vi "InvertedCalculationProjectionAngleOffset.vi"(6 "Y offset":dbl, 7 "X offset":dbl, 8 "RangeX":dbl, 9 "Angle":dbl, 10 "Height":dbl) -> (3 "Width":dbl)   [LabVIEW 2016]
panel:
  out "ResultX":dbl
  out "ResultY":dbl
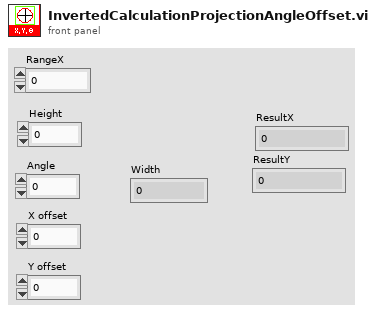
[diagram p1: front panel]
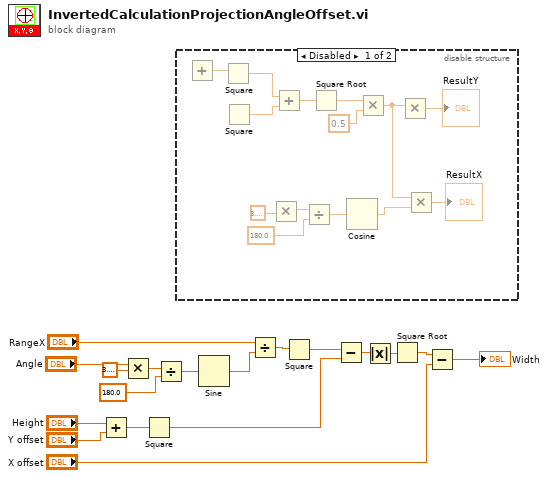
[diagram p0: block diagram]
diagram:
  n1 = Add(x="Height", y="Y offset") -> (x+y=w9:dbl)
  n2 = Multiply(x="Angle", y=3.141592653589793) -> (x*y=w4:dbl)
  n3 = Square(x=w9) -> (x^2=w8:dbl)
  n4 = Divide(x=w4, y=180.0) -> (x/y=w17:dbl)
  n5 = disable-structure shown="Disabled" {
    frame Disabled {
      n6 = Add() -> (x+y=w26:dbl)  [unwired: 2 in]
      n7 = Square(x=w26) -> (x^2=w32:dbl)
      n8 = Square() -> (x^2=w31:dbl)  [unwired: 1 in]
      n9 = Multiply(y=3.141592653589793) -> (x*y=w23:dbl)  [unwired: 1 in]
      n10 = Add(x=w32, y=w31) -> (x+y=w30:dbl)
      n11 = Divide(x=w23, y=180.0) -> (x/y=w25:dbl)
      n12 = Square Root(x=w30) -> (sqrt(x)=w28:dbl)
      n13 = Cosine(x=w25) -> (cos(x)=w20:dbl)
      n14 = Multiply(x=w28, y=0.5) -> (x*y=w21:dbl)
      n15 = Multiply(x=w21) -> (x*y=→"ResultY":dbl)  [unwired: 1 in]
      n16 = Multiply(x=w21, y=w20) -> (x*y=→"ResultX":dbl)
    }
    frame Enabled {
    }
  }
  n17 = Sine(x=w17) -> (sin(x)=w14:dbl)
  n18 = Divide(x="RangeX", y=w14) -> (x/y=w13:dbl)
  n19 = Square(x=w13) -> (x^2=w12:dbl)
  n20 = Subtract(x=w12, y=w8) -> (x-y=w2:dbl)
  n21 = Absolute Value(x=w2) -> (abs(x)=w1:dbl)
  n22 = Square Root(x=w1) -> (sqrt(x)=w7:dbl)
  n23 = Subtract(x=w7, y="X offset") -> (x-y=→"Width":dbl)
